vi "ControlProcessWindow.vi"(0 "reference in":refnum<class "ZeroMQ.lvclass">, 2 "ShowProcessWindow":bool, 5 "error in (no error)":errorcluster) -> (14 "reference out":refnum<class "ZeroMQ.lvclass">, 19 "error out":errorcluster)   [LabVIEW 2018, in "ZeroMQ.lvclass"]
doc: "Can show or hide the process window, which will show you debug and execution information of the messages coming by."
uses:
  ZeroMQ.lvclass
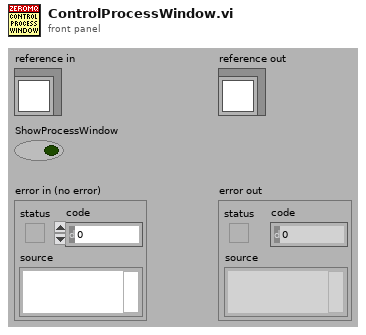
[diagram p1: front panel]
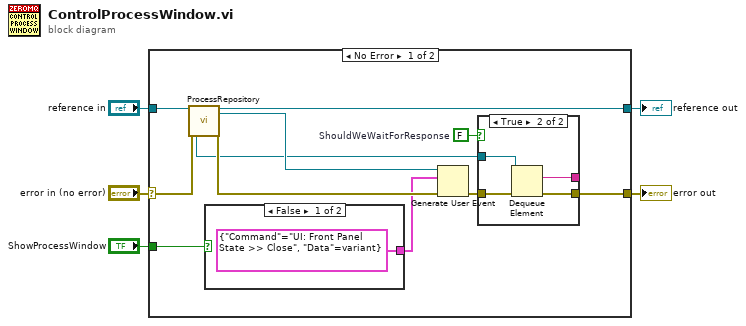
[diagram p0: block diagram]
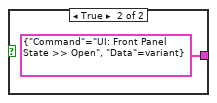
[diagram p2: hidden frame]
diagram:
  n1 = case shown="No Error" "error in (no error)" {
    selector: "error in (no error)" -> [w9 w25]
    tunnel: [w11 w25] -> w1
    tunnel: [w15 w24] -> w4
    tunnel: "reference in" -> [w16 w24]
    tunnel: "ShowProcessWindow" -> [w7 _]
    frame No Error {
      w6 = FALSE  # ShouldWeWaitForResponse
      n2 = call "ProcessRepository.vi"("reference in"=w16, "error in (no error)"=w9) -> ("QueueFromProcess"=w10:refnum<queue>, "reference out"=w15:refnum<class "ZeroMQ.lvclass">, "EventsToProcess"=w14:refnum<user-event>, "error out"=w12:errorcluster)  [unwired: 10 in, 4 out]
      n3 = case shown="False" w7 {
        tunnel: [cluster{"Command":string, "Data":variant} {"Command"="UI: Front Panel State >> Close", "Data"=variant} ("MessageToProcess") cluster{"Command":string, "Data":variant} {"Command"="UI: Front Panel State >> Open", "Data"=variant} ("MessageToProcess")] -> w8
        frame False {
        }
        frame True {
        }
      }
      n4 = Generate User Event(user event=w14, event data cluster=w8, error in=w12) -> (error out=w13:errorcluster)  [unwired: 1 in, 1 out]
      n5 = case shown="True" w6 {
        tunnel: w13 -> [w19 w23]
        tunnel: [_ w22] -> _
        tunnel: [w19 w21] -> w11
        tunnel: w10 -> [_ w20]
        frame False {
        }
        frame True {
          n6 = Dequeue Element(queue=w20, error in (no error)=w23) -> (element=w22:string, error out=w21:errorcluster)  [unwired: 1 in, 2 out]
        }
      }
    }
    frame Error {
    }
  }
  "error out" <- w1
  "reference out" <- w4
